vi "CheckWindSetpointFile.vi"(2 "File Name":string, 3 "Setpoints In":dbl[][](array[numeric])) -> (0 "Read error":string, 1 "Setpoints Out":dbl[][](array[numeric]))   [LabVIEW 2018]
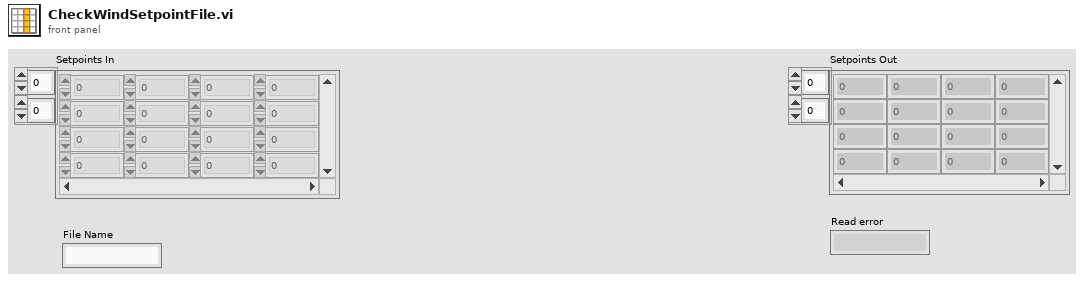
[diagram p1: front panel]
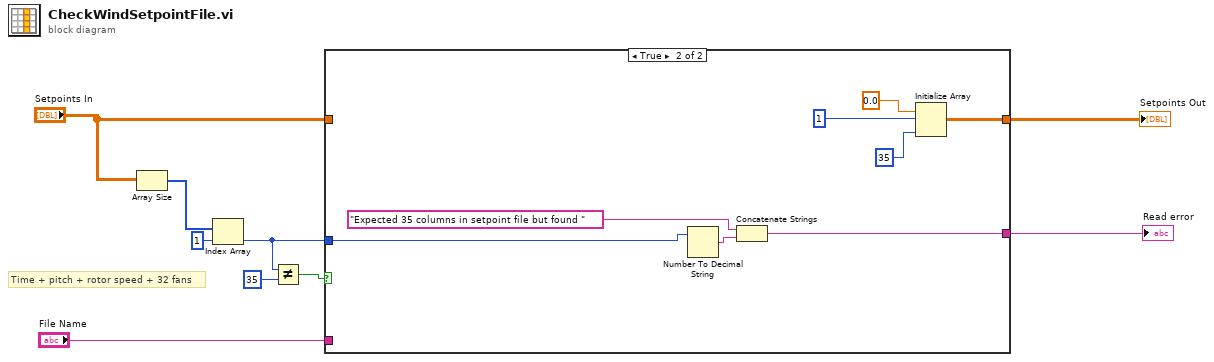
[diagram p0: block diagram]
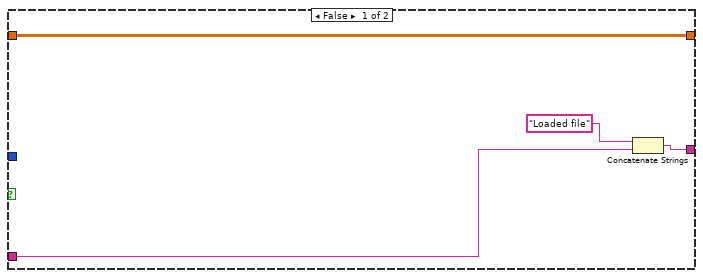
[diagram p2: hidden frame]
diagram:
  # "Time + pitch + rotor speed + 32 fans"
  n1 = Array Size(array="Setpoints In") -> (size(s)=w9:i32[])
  n2 = Index Array(array=w9, index=1) -> (element=w6:i32)
  n3 = Not Equal?(x=w6, y=35) -> (x != y?=w5:bool)
  n4 = case shown="True" w5 {
    tunnel: w6 -> [_ w20]
    tunnel: [w12 w18] -> w2
    tunnel: "Setpoints In" -> [w13 _]
    tunnel: [w13 w14] -> w3
    tunnel: "File Name" -> [w10 _]
    frame False {
      n5 = Concatenate Strings("Loaded file" ("string"), w10) -> (w12:string)
    }
    frame True {
      n6 = Number To Decimal String(number=w20) -> (decimal integer string=w19:string)  [unwired: 1 in]
      n7 = Concatenate Strings("Expected 35 columns in setpoint file but found ", w19) -> (w18:string)
      n8 = Initialize Array(0.0 ("element"), 1 ("dimension size"), 35 ("dimension size")) -> (w14:dbl[][])
    }
  }
  "Setpoints Out" <- w3
  "Read error" <- w2
